vi "DSS.vi"(0 "VISAリソース名":refnum<visa-resource-name>, 5 "文字列待機 (350 ms)":u16=350, 11 "error in (no error)":errorcluster caption="エラー入力（エラーなし）") -> (4 "VISAリソース名（出力）":refnum<visa-resource-name>, 6 "Status":string, 8 "Coil":string, 10 "Amplitude":i16, 13 "Ramp":i8, 14 "Delay":i8, 15 "error out":errorcluster caption="エラー出力")   [LabVIEW 2017]
panel:
  out "文字列":string
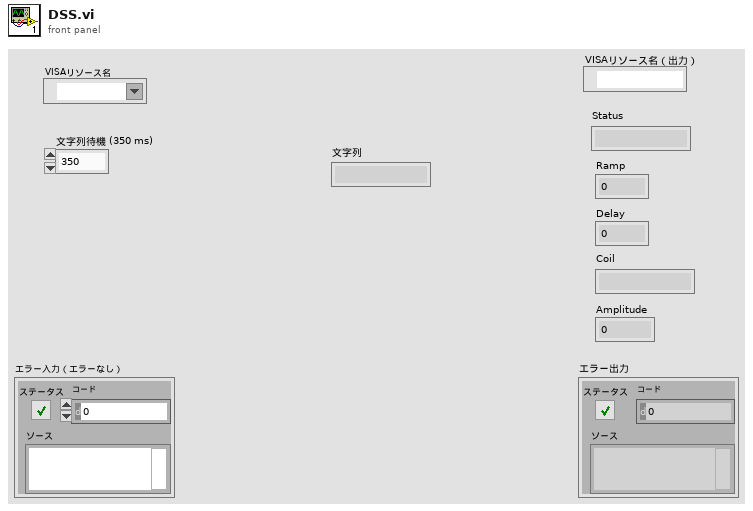
[diagram p1: front panel]
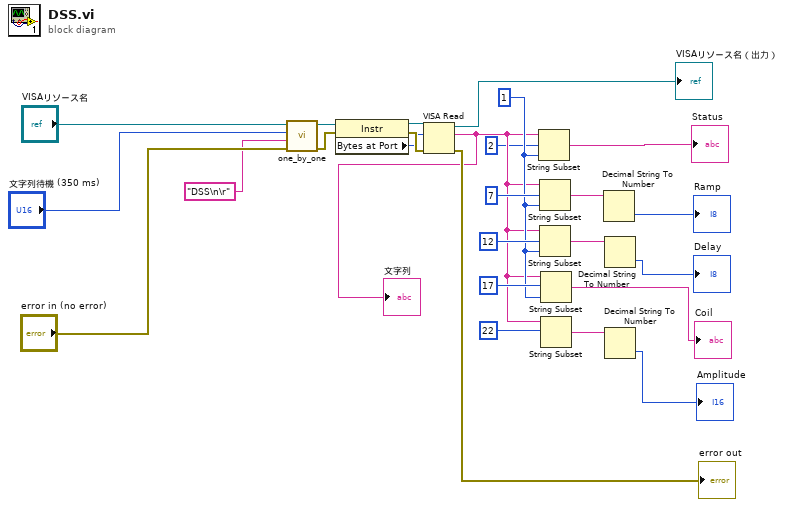
[diagram p0: block diagram]
diagram:
  w14 = 1
  n1 = call "one_by_one.vi"("error in (no error)"="error in (no error)", "入力文字"="DSS\n\r", "待機 (200ms)"="文字列待機 (350 ms)", "VISAリソース名"="VISAリソース名") -> ("error out"=w18:errorcluster, "VISAリソース名出力"=w19:refnum<visa-resource-name>)  [unwired: 6 in]
  n2 = property class="Instr"(reference=w19, error in=w18) -> (reference out=w20:refnum<visa-resource-name>, error out=w22:errorcluster, "Bytes at Port"=w21:u32)
  n3 = VISA Read(VISA resource name=w20, byte count=w21, error in (no error)=w22) -> (VISA resource name out=→"VISAリソース名（出力）":refnum<visa-resource-name>, read buffer=w3:string, error out=→"error out":errorcluster)  [unwired: 1 out]
  "文字列" <- w3
  n4 = String Subset(string=w3, offset (0)=2, length (rest)=w14) -> (substring=→"Status":string)
  n5 = String Subset(string=w3, offset (0)=7, length (rest)=w14) -> (substring=w13:string)
  n6 = String Subset(string=w3, offset (0)=12, length (rest)=w14) -> (substring=w12:string)
  n7 = String Subset(string=w3, offset (0)=17, length (rest)=w14) -> (substring=→"Coil":string)
  n8 = String Subset(string=w3, offset (0)=22) -> (substring=w11:string)  [unwired: 1 in]
  n9 = Decimal String To Number(string=w13) -> (number=→"Ramp":i32)  [unwired: 2 in, 1 out]
  n10 = Decimal String To Number(string=w12) -> (number=→"Delay":i32)  [unwired: 2 in, 1 out]
  n11 = Decimal String To Number(string=w11) -> (number=→"Amplitude":i32)  [unwired: 2 in, 1 out]
